vi "mic test.vi"() -> ()   [LabVIEW 2023]
panel:
  in  "Duration (s)":dbl=4.5
  in  "Sample rate (Hz)":dbl=58000.0
  out "Data":dynamicdata(graph)
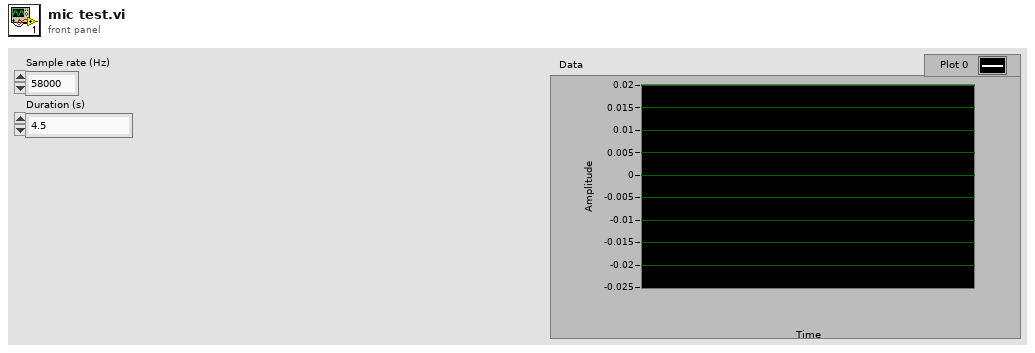
[diagram p1: front panel]
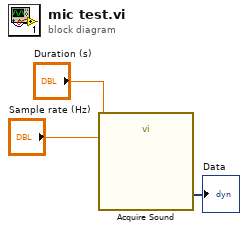
[diagram p0: block diagram]
diagram:
  n1 = call "Acquire Sound"("Duration (s)"="Duration (s)", "Sample rate (Hz)"="Sample rate (Hz)") -> ("Data"=→"Data":dynamicdata)  [unwired: 16 in, 1 out]
